vi "TDC_DAQV23_Paralled_muon_temp.vi"(8 "error in (no error)":errorcluster, 9 "stop":bool, 10 "save data":bool=TRUE, 11 "SMA mode":bool) -> (0 "error out 3":errorcluster, 2 "appended path":path=path "D:/tdc/2017/test_20241012_085406.csv", 3 "rate":dbl=30.96114492240285)   [LabVIEW 2017]
uses:
  gloabal.vi
  <vilib>/Utility/file.llb/Write Delimited Spreadsheet (DBL).vi
  <vilib>/Utility/file.llb/Write Delimited Spreadsheet (I64).vi
panel:
  in  "timeout":dbl=120.0 format="%#_13g"
  in  "GPS":bool
  out "name (unnamed)":string
  out "x+y":u64
  out "ip":string[](array[string])
  out "error out 4":errorcluster
  in  "timeout (ms) 2":i32=10000
  in  "address":string[](array[string])=["192.168.10.23", "192.168.10.22"]
  out "substring 4":string
  out "substring 3":string
  out "hex integer string":string="07E8"
  out "Year":string="2024"
  out "substring 2":string
  out "substring":string
  in  "factor":i32=128
  in  "displayCR":bool=TRUE
  in  "Counter Setting":dbl=100000.0 format="%#_13g"
  in  "replace dat":bool
  in  "append csv":bool=TRUE
  out "number":u32=22
  out "element":string
  out "fine":u64=330 format="%x"
  in  "UDP Config":bool=TRUE
  in  "data  path":path=path "D:/tdc/2017"
  out "cal 2":u64[](graph)
  in  "Thresholds (mV)":u16[](array[numeric])=[580, 580, 580, 580, 600, 600, 600, 600, 580, 580, 600, 600, 600, 600, 600, 600, 580, 580, 600, 600, 600, 600, 600, 600, 580, 580, 600, 600, 600, 600, 600, 600]
  out "error out 2":errorcluster
  in  "display":bool=TRUE
  in  "Thresholds":u16=600
  in  "one key for threshold":bool=TRUE
  in  "RST":bool
  in  "通道数量":i32=64
  out "Cal Table":u32[](array[numeric])=[0, 0, 0, 0, 0, 0, 0, 0, 0, 0, 0, 0, 0, 0, 53560, 53560, 0, 0, 0, 0, 0, 0, 0, 0, 0, 0, 0, 0, 0, 0, 0, 0, 0, 0, 0, 0, 0, 0, 0, 0, 0, 0, 0, 0, 0, 0, 0, 0, 0, 0, 0, 0, 0, 0, 0, 0, 0, 0, 0, 0, 0, 0, 0, 0, 0, 0, 0, 0, 0, 0, 0, 0, 0, 0, 0, 0, 0, 0, 0, 0, 0, 0, 0, 0, 0, 0, 0, 0, 0, 0, 0, 0, 0, 0, 0, 0, 0, 0, 0, 0, 0, 0, 0, 0, 0, 0, 0, 0, 0, 0, 0, 0, 0, 0, 0, 0, 0, 0, 53560, 53560, 0, 0, 0, 0, 0, 0, 0, 0]
  in  "channel for cal":i32=61
  out "channel number":u64
  out "Calibration Counter":i32=53569
  out "cal":u32[](graph)
  out "error out":errorcluster
  in  "filename":string="test"
  in  "Events":i32=110000 min=1
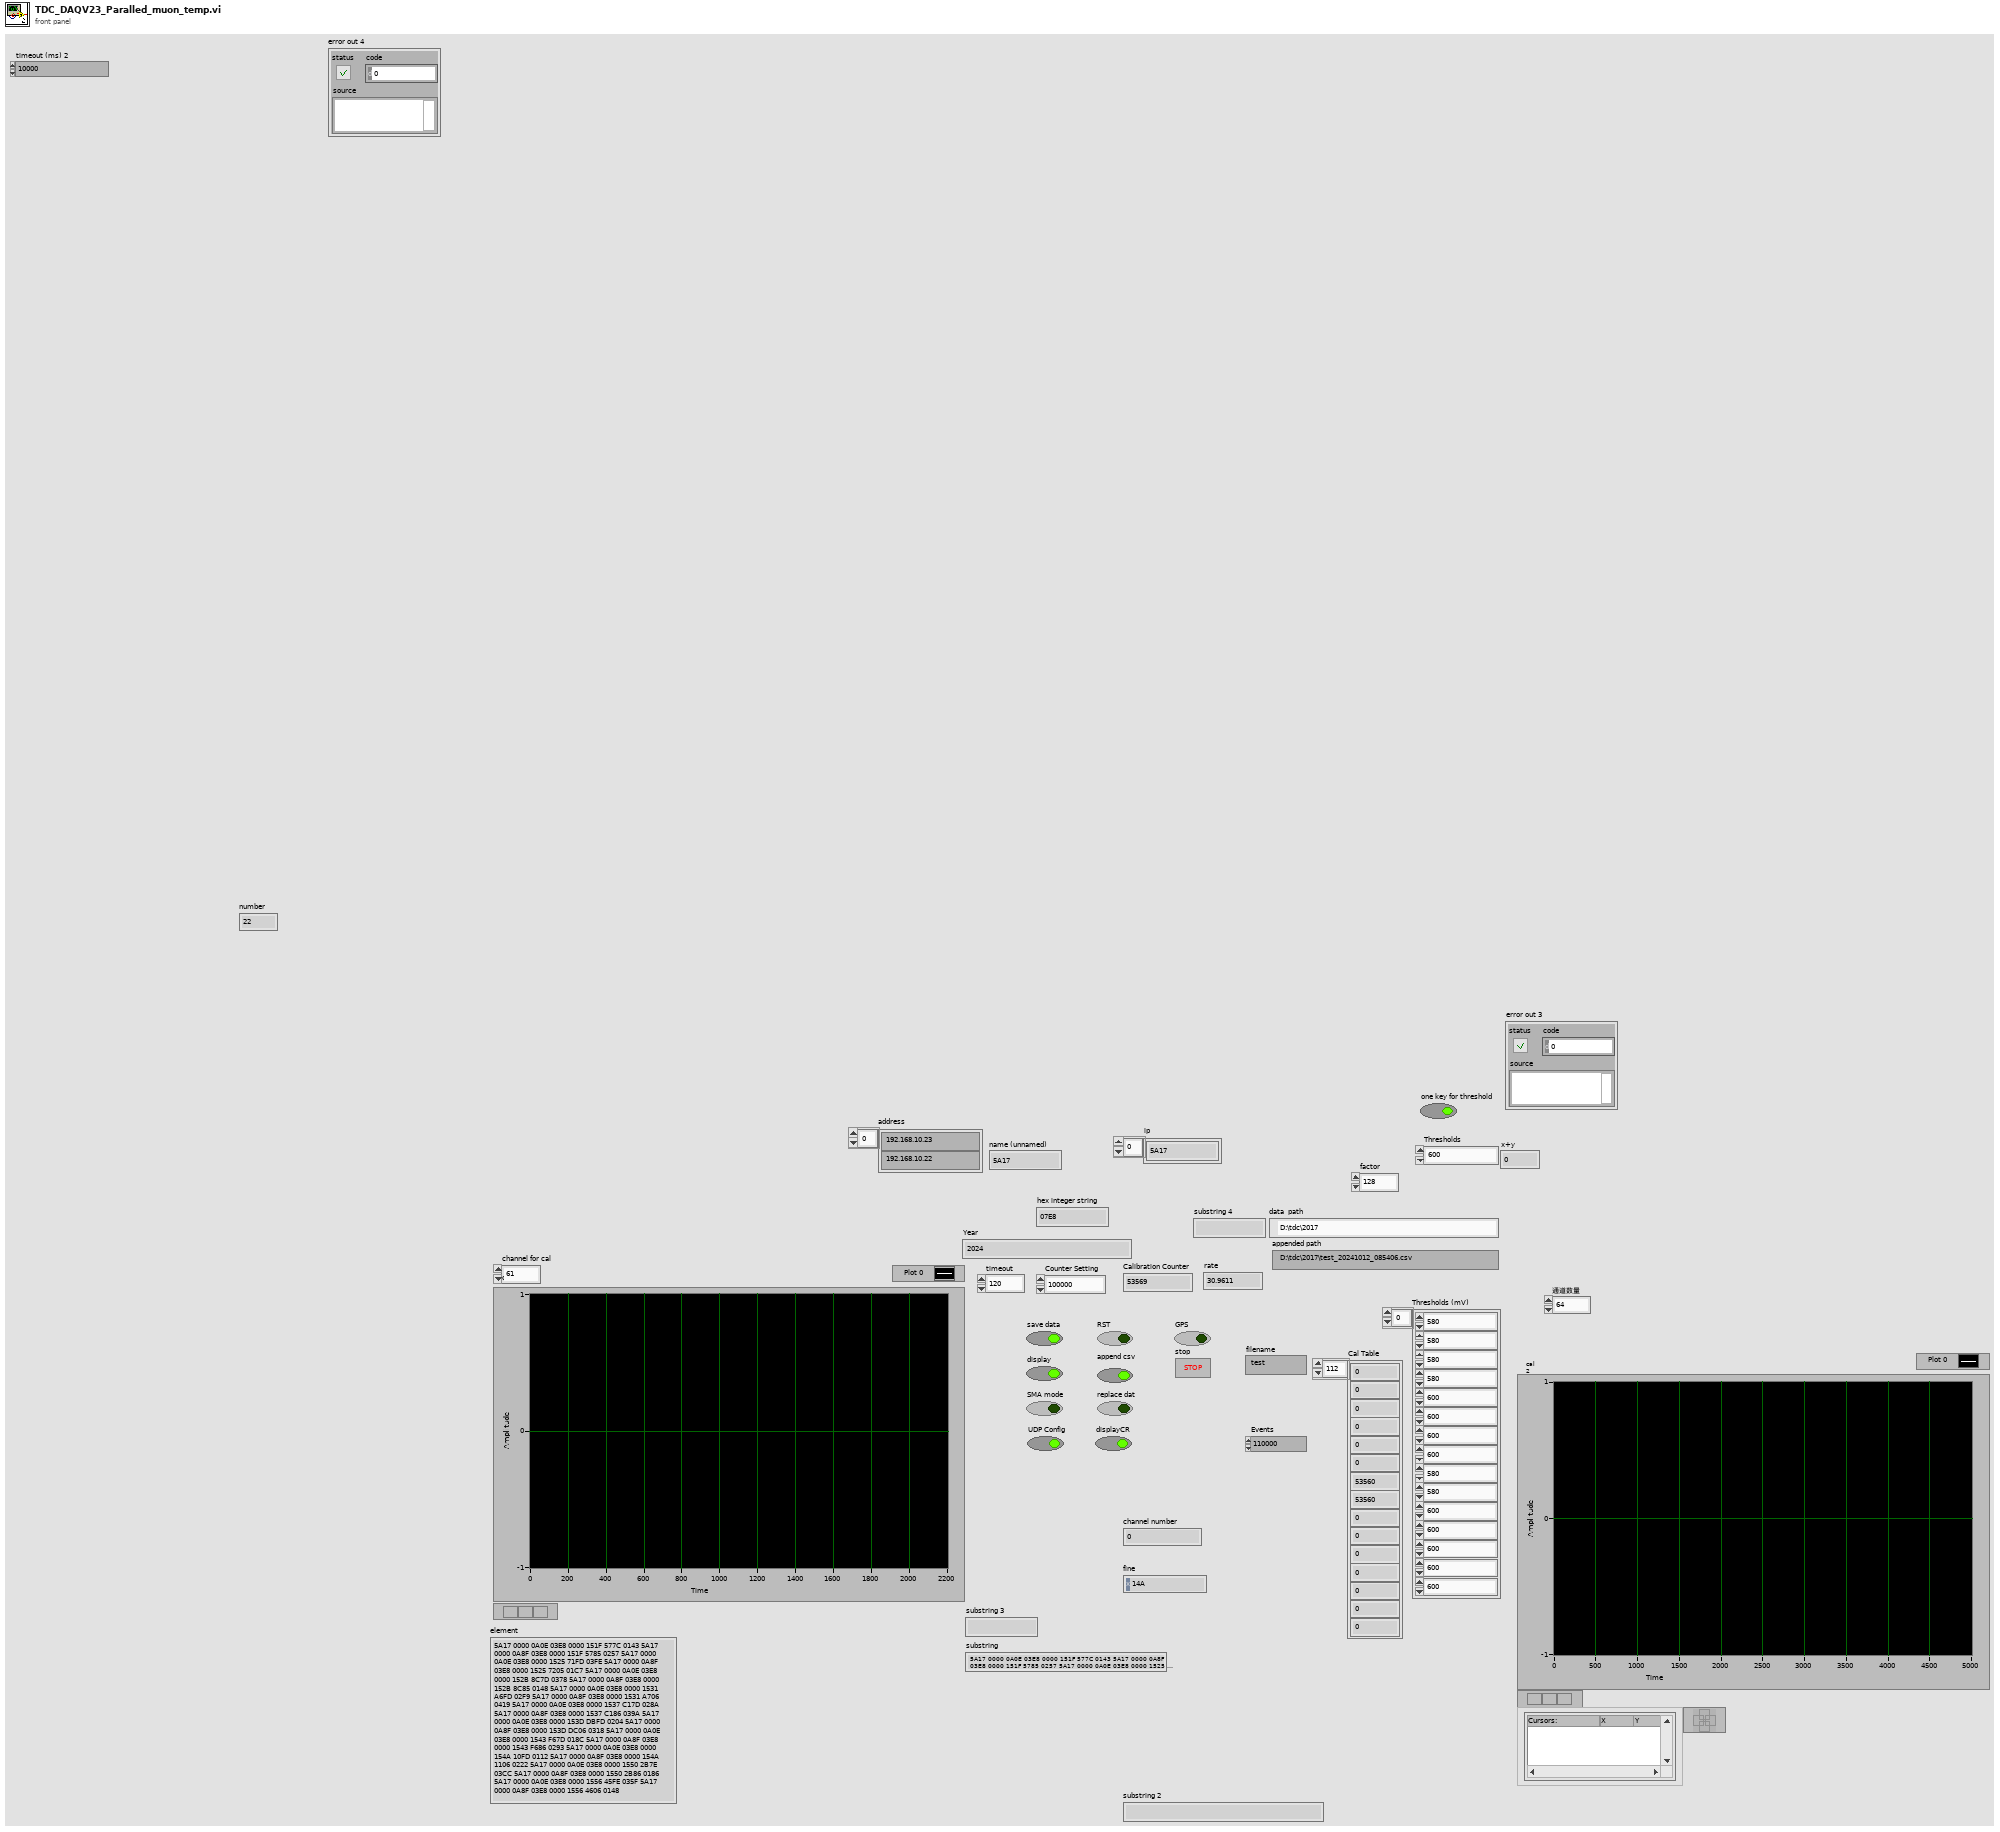
[diagram p1: front panel]
types:
  T1 = enum16{"open", "replace", "create", "open or create", "replace or create", "replace or create with confirmation"}
  T2 = enum16{"big-endian, network order", "native, host order", "little-endian"}
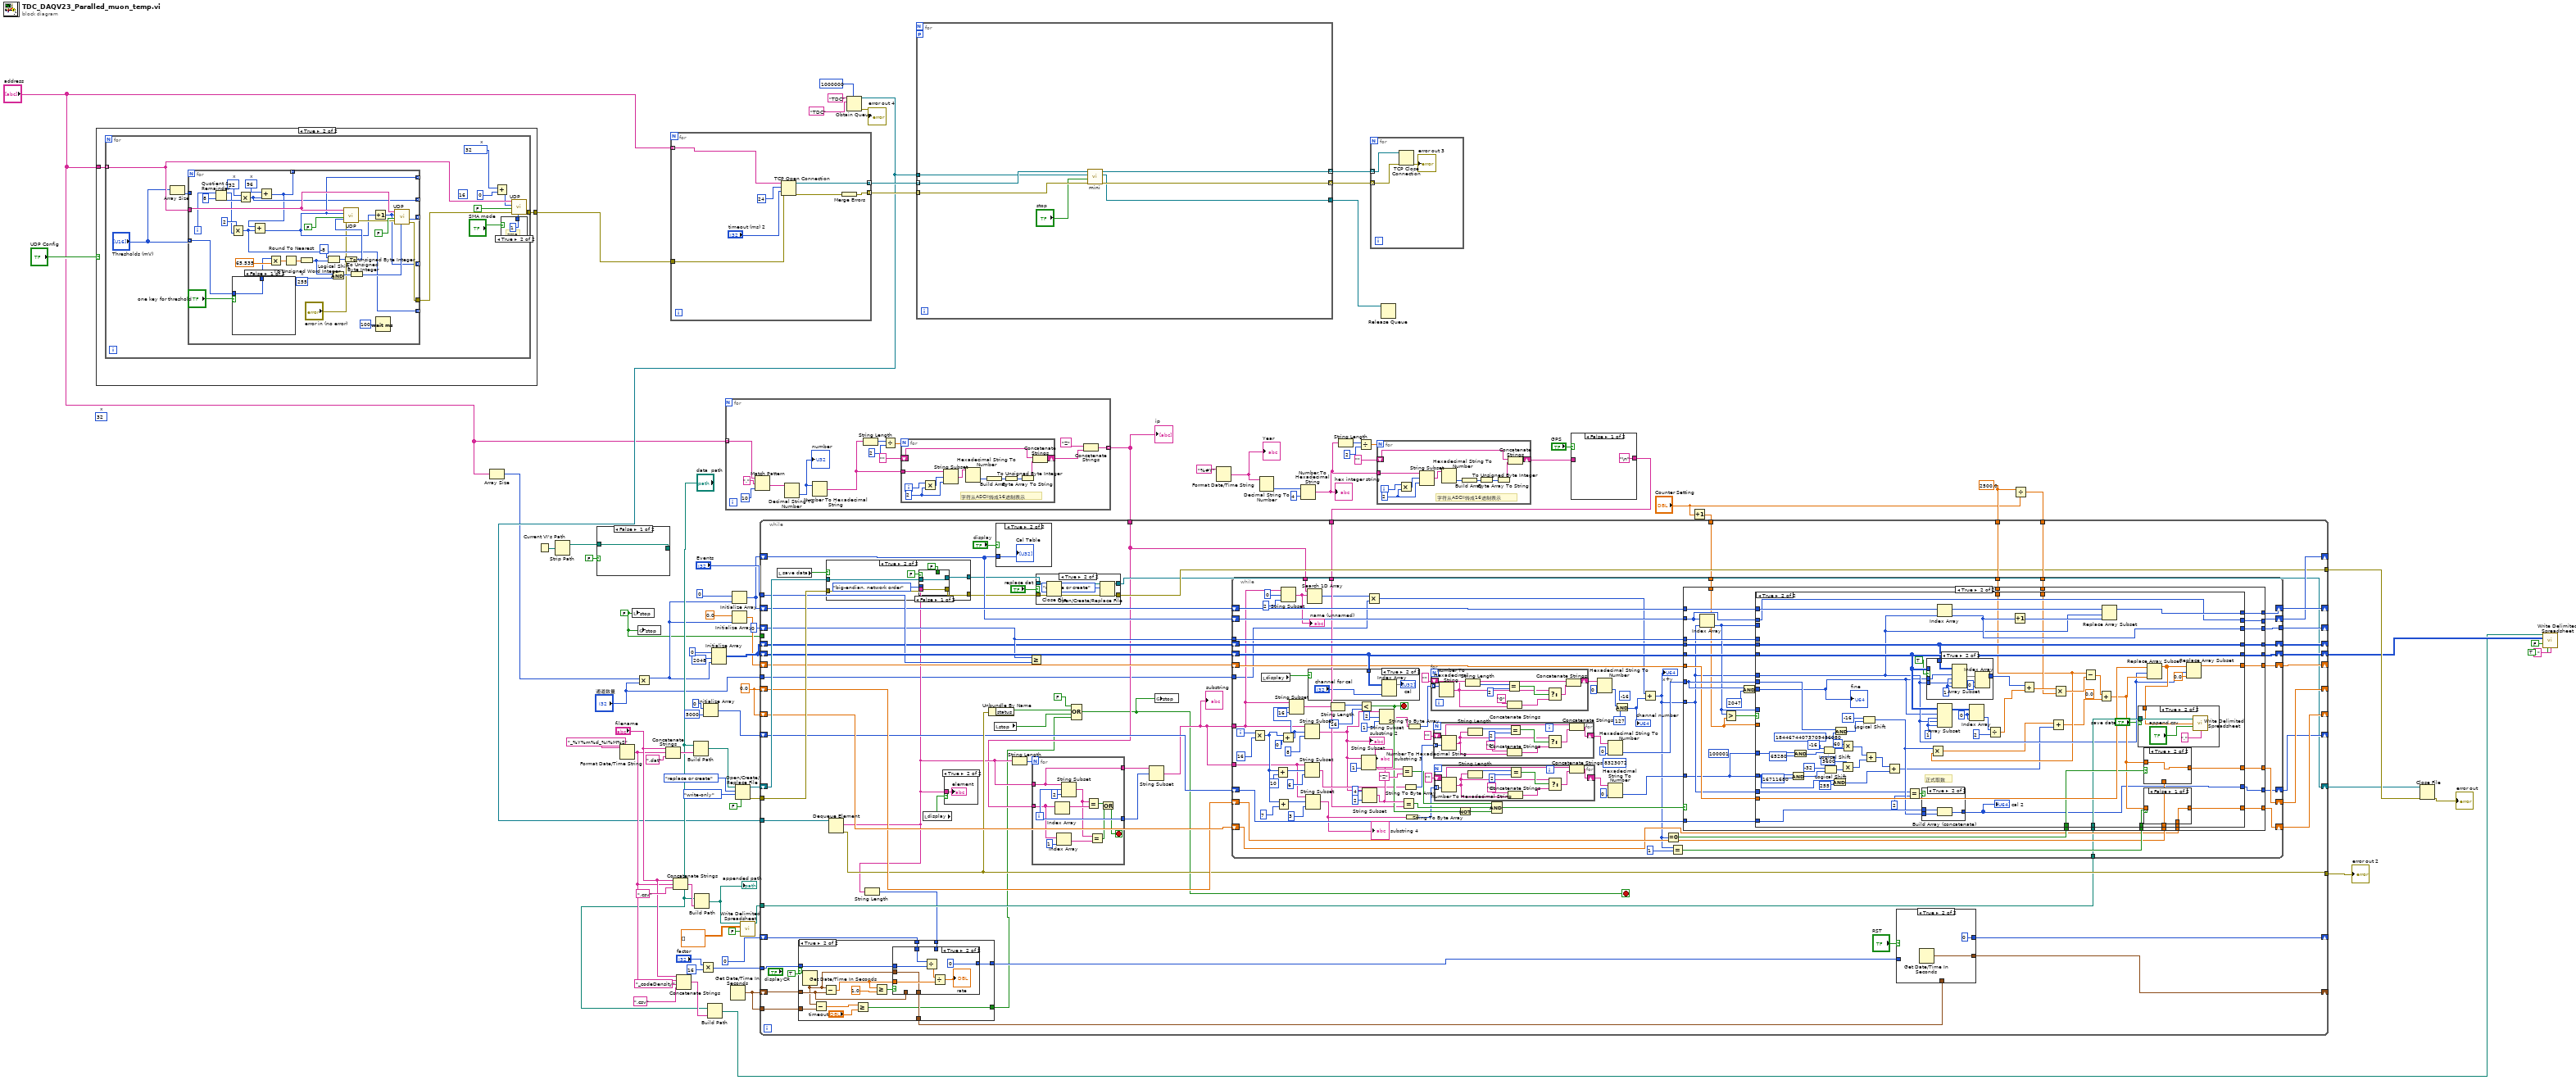
[diagram p0: block diagram]
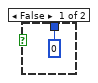
[diagram p4: hidden frame]
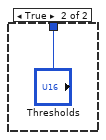
[diagram p5: hidden frame]
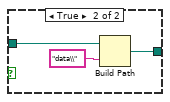
[diagram p6: hidden frame]
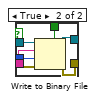
[diagram p9: hidden frame]
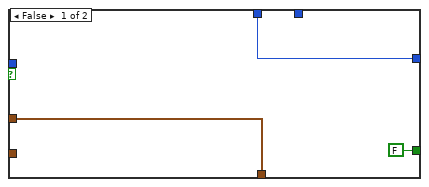
[diagram p11: hidden frame]
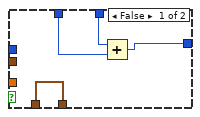
[diagram p12: hidden frame]
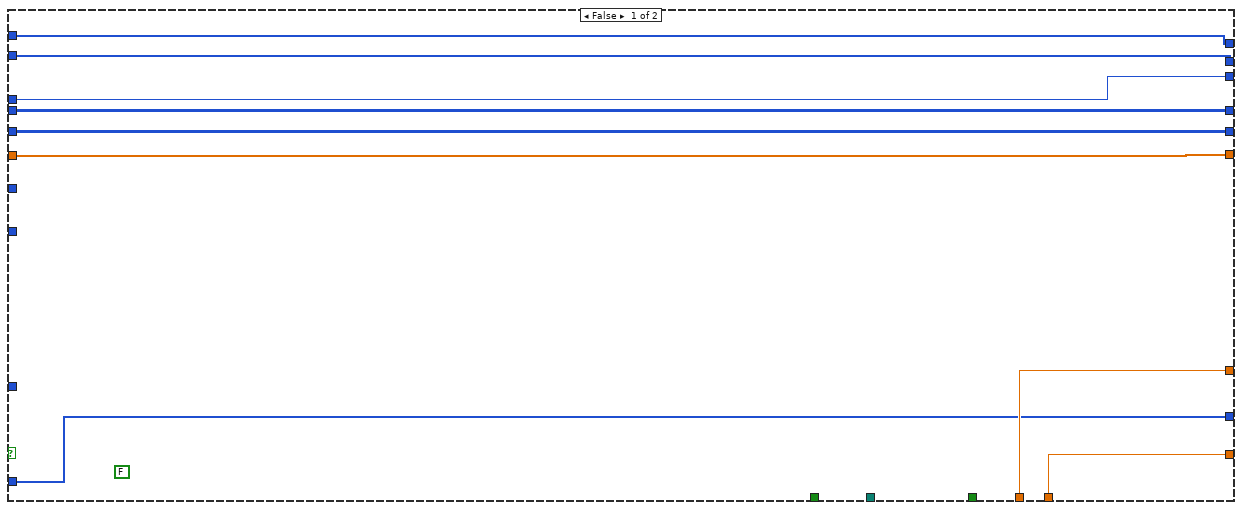
[diagram p16: hidden frame]
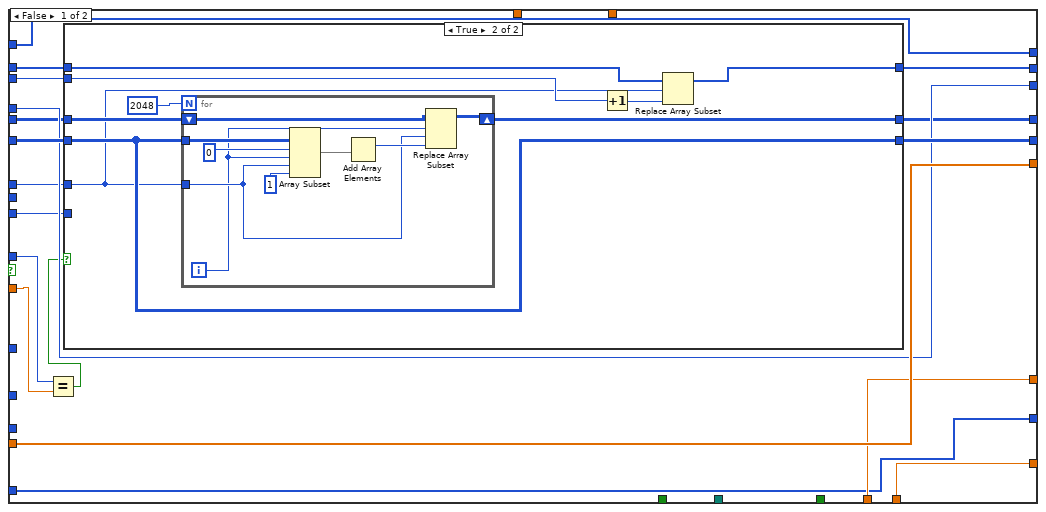
[diagram p17: hidden frame]
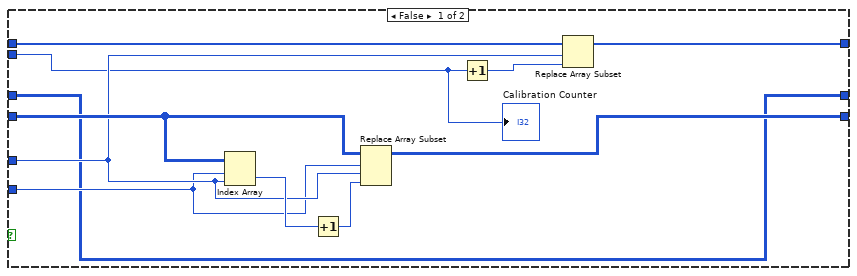
[diagram p18: hidden frame]
diagram:
  w40 = 2500.0 ("x")
  (unwired) u16 32  # x
  w3 = FALSE ("stop")
  w64 = 0.0
  n1 = case shown="True" "UDP Config" {
    tunnel: "address" -> [_ w87]
    tunnel: [_ w86] -> w13
    frame False {
    }
    frame True {
      n2 = for {
        tunnel: w87 -> [w98] mode=indexing
        tunnel: [w95] -> w86
        (unwired) u32 16 ("Address")
        w89 = u16 32  # x
        n3 = Array Size(array="Thresholds (mV)") -> (size(s)=w92:i32)
        n4 = for {
          tunnel: w98 -> [w128]
          tunnel: "Thresholds (mV)" -> [w114] mode=indexing
          tunnel: [w122] -> _ mode=indexing
          tunnel: [w117] -> w96
          tunnel: w92 -> [_]
          tunnel: [w108] -> _ mode=indexing
          tunnel: [w107] -> _ mode=indexing
          tunnel: [w106] -> _ mode=indexing
          tunnel: [w105] -> _ mode=indexing
          tunnel: [w104] -> _ mode=indexing
          i -> [w109]
          w110 = u16 96  # x
          w111 = u16 32  # x
          w124 = u16 255  # x
          n5 = Quotient & Remainder(x=w109, y=8) -> (x-y*floor(x/y)=w103:i32, floor(x/y)=w112:i32)
          n6 = Multiply(x=2, y=w103) -> (x*y=w104:i32)
          n7 = case shown="False" "one key for threshold" {
            tunnel: [w134 "Thresholds"] -> w115
            tunnel: w114 -> [w134 _]
            frame False {
            }
            frame True {
            }
          }
          n8 = Multiply(x=w111, y=w112) -> (x*y=w106:i32)
          n9 = Add(x=w110, y=w106) -> (x+y=w105:i32)
          n10 = Add(x=w105, y=w104) -> (x+y=w108:i32)
          n11 = Multiply(x=w115, y=65.535) -> (x*y=w131:dbl)
          n12 = Round To Nearest(number=w131) -> (nearest integer value=w129:dbl)
          n13 = To Unsigned Word Integer(number=w129) -> (unsigned 16bit integer=w119:u16)
          n14 = Logical Shift(y=i16 -8, x=w119) -> (x << y=w126:u16)
          n15 = And(x=w119, y=w124) -> (x .and. y?=w123:u16)
          n16 = To Unsigned Byte Integer(number=w126) -> (unsigned 8bit integer=w125:u8)
          n17 = call "UDP.vi"("In"=w125, "error in (no error)"="error in (no error)", "Read (TRUE)"=FALSE, "Address"=w108, "IP address"=w128) -> ("error out"=w118:errorcluster)  [unwired: 4 in, 1 out]
          n18 = To Unsigned Byte Integer(number=w123) -> (unsigned 8bit integer=w121:u8)
          n19 = Increment(x=w108) -> (x+1=w107:i32)
          n20 = Wait (ms)(milliseconds to wait=u32 100) -> ()  [unwired: 1 out]
          n21 = call "UDP.vi"("In"=w121, "error in (no error)"=w118, "Read (TRUE)"=FALSE, "Address"=w107, "IP address"=w128) -> ("error out"=w117:errorcluster, "Out"=w122:u8)  [unwired: 4 in]
        }
        n22 = Add(x=w89, y=u32 0 ("Address")) -> (x+y=w88:u32)
        n23 = case shown="True" "SMA mode" {
          tunnel: [u8 0 ("In") u8 1 ("In")] -> w94
          frame False {
          }
          frame True {
            # "sma"
          }
        }
        n24 = call "UDP.vi"("In"=w94, "error in (no error)"=w96, "Read (TRUE)"=FALSE, "Address"=w88, "IP address"=w98) -> ("error out"=w95:errorcluster)  [unwired: 4 in, 1 out]
      }
    }
  }
  n25 = Array Size(array="address") -> (size(s)=w8:i32)
  n26 = Current VI's Path() -> (path=w80:path)
  n27 = Strip Path(path=w80) -> (stripped path=w79:path)  [unwired: 1 out]
  n28 = case shown="False" FALSE {
    tunnel: w79 -> [w136 w138]
    tunnel: [w136 w137] -> _
    frame False {
    }
    frame True {
      n29 = Build Path(base path=w138, name or relative path="data\\") -> (appended path=w137:path)
    }
  }
  n30 = Format Date/Time String(time format string (%c)="_%Y%m%d_%I%M%S") -> (date/time string=w57:string)  [unwired: 2 in]
  n31 = local write "stop"(w3) -> ()
  n32 = Multiply(x=w8, y="通道数量") -> (x*y=w10:i32)
  n33 = global write "gloabal.vi" "stop"(w3) -> ()
  n34 = Concatenate Strings("filename", w57, ".dat") -> (w78:string)
  n35 = for {
    tunnel: "address" -> [w144] mode=indexing
    tunnel: [w143] -> w22 mode=indexing
    tunnel: [w141] -> w21 mode=indexing
    tunnel: w13 -> [w140]
    n36 = TCP Open Connection(address=w144, remote port or service name=u16 24 ("port"), timeout ms (60000)="timeout (ms) 2", error in (no error)=w140) -> (connection ID=w143:refnum<k5>, error out=w142:errorcluster)  [unwired: 1 in]
    n37 = Merge Errors(w142) -> (w141:errorcluster)
  }
  n38 = Concatenate Strings("filename", w57, ".csv") -> (w66:string)
  n39 = Concatenate Strings("filename", w57, "_codeDensity" ("string"), ".csv") -> (w54:string)
  n40 = Build Path(base path="data  path", name or relative path=w78) -> (appended path=w77:path)
  n41 = Build Path(base path="data  path", name or relative path=w66) -> (appended path=w2:path)
  "appended path" <- w2
  n42 = Multiply(x="factor", y=16) -> (x*y=w33:i32)
  n43 = Initialize Array(u32 0 ("element"), 5000 ("dimension size")) -> (w45:u32[])
  n44 = Build Path(base path="data  path", name or relative path=w54) -> (appended path=w51:path)
  n45 = Initialize Array(u32 0 ("element"), 2048 ("dimension size"), w10) -> (w63:u32[][])
  n46 = for {
    tunnel: [w148] -> w9 mode=indexing
    tunnel: "address" -> [w147] mode=indexing
    n47 = Match Pattern(string=w147, regular expression="." ("search string"), offset (0)=10) -> (after substring=w152:string)  [unwired: 3 out]
    n48 = Decimal String To Number(string=w152) -> (number=w151:i32)  [unwired: 2 in, 1 out]
    "number" <- w151
    n49 = Number To Hexadecimal String(2:w151) -> (0:w150:string)  [unwired: 1 in]
    n50 = String Length(string=w150) -> (length=w157:i32)
    n51 = Divide(x=w157, y=2) -> (x/y=w158:dbl)
    n52 = for {
      N: w158 -> [_]
      shift-right: [w170] -> w149
      shift-left: "" ("format string") -> [w169]
      tunnel: w150 -> [w160]
      i -> [w168]
      w162 = 2 ("y")
      # "字符从ASCII转成16进制表示"
      n53 = Multiply(x=w168, y=w162) -> (x*y=w161:i32)
      n54 = String Subset(string=w160, offset (0)=w161, length (rest)=w162) -> (substring=w163:string)
      n55 = Hexadecimal String To Number(string=w163) -> (number=w167:u32)  [unwired: 2 in, 1 out]
      n56 = Build Array(w167) -> (w166:u32[])
      n57 = To Unsigned Byte Integer(number=w166) -> (unsigned 8bit integer=w165:u8[])
      n58 = Byte Array To String(unsigned byte array=w165) -> (string=w164:string)
      n59 = Concatenate Strings(w169, w164) -> (w170:string)
    }
    n60 = Concatenate Strings("Z", w149) -> (w148:string)
  }
  "ip" <- w9
  n61 = Get Date/Time In Seconds() -> (seconds since 1Jan1904=w1:timestamp)
  n62 = Initialize Array(u32 0 ("element"), w10) -> (w65:u32[])
  n63 = Initialize Array(0.0, w10) -> (w47:dbl[])
  n64 = Open/Create/Replace File(file path (use dialog)=w77, operation (0:open)=T1."replace or create", access (0:read/write)=enum16{"read/write", "read-only", "write-only"}."write-only", disable buffering (F)=FALSE) -> (refnum out=w82:refnum<file>, error out=w81:errorcluster)  [unwired: 2 in, 1 out]
  n65 = call-poly <vilib>:"Write Delimited Spreadsheet.vi"("file path (dialog if empty)"=w2, "2D data"=dbl[][] [], "append to file? (new file:F)"=FALSE) -> ("new file path (Not A Path if cancelled)"=w61:path)  [unwired: 11 in, 1 out]
  n66 = Obtain Queue(max queue size (-1, unlimited)=1000000, name (unnamed)="TDC", element data type="TDC" ("name (unnamed)")) -> (queue out=w12:refnum<queue>, error out=→"error out 4":errorcluster)  [unwired: 2 in, 1 out]
  n67 = for {
    tunnel: w22 -> [w177] mode=indexing
    tunnel: w21 -> [w176] mode=indexing
    tunnel: [w175] -> w20 mode=indexing
    tunnel: [w174] -> w19 mode=indexing
    workers-P: _ -> [_]
    tunnel: w12 -> [w173]
    tunnel: [w172] -> w14
    n68 = call "mini.vi"("error in (no error)"=w176, "stop"="stop", "queue out 2"=w173, "connection ID 2"=w177) -> ("error out 3"=w174:errorcluster, "queue out"=w172:refnum<queue>, "connection ID"=w175:refnum<k5>)  [unwired: 5 in]
  }
  n69 = Format Date/Time String(time format string (%c)="%#Y") -> (date/time string=w30:string)  [unwired: 2 in]
  "Year" <- w30
  n70 = Decimal String To Number(string=w30) -> (number=w29:i32)  [unwired: 2 in, 1 out]
  n71 = Number To Hexadecimal String(1:i16 4 ("width (-)"), 2:w29) -> (0:w23:string)
  "hex integer string" <- w23
  n72 = String Length(string=w23) -> (length=w25:i32)
  n73 = Divide(x=w25, y=2) -> (x/y=w26:dbl)
  n74 = for {
    tunnel: w20 -> [w180] mode=indexing
    tunnel: w19 -> [w179] mode=indexing
    n75 = TCP Close Connection(connection ID=w180, error in (no error)=w179) -> (error out=→"error out 3":errorcluster)  [unwired: 1 in, 1 out]
  }
  n76 = for {
    N: w26 -> [_]
    shift-right: [w191] -> w5
    shift-left: "" ("format string") -> [w190]
    tunnel: w23 -> [w181]
    i -> [w189]
    w183 = 2 ("y")
    # "字符从ASCII转成16进制表示"
    n77 = Multiply(x=w189, y=w183) -> (x*y=w182:i32)
    n78 = String Subset(string=w181, offset (0)=w182, length (rest)=w183) -> (substring=w184:string)
    n79 = Hexadecimal String To Number(string=w184) -> (number=w188:u32)  [unwired: 2 in, 1 out]
    n80 = Build Array(w188) -> (w187:u32[])
    n81 = To Unsigned Byte Integer(number=w187) -> (unsigned 8bit integer=w186:u8[])
    n82 = Byte Array To String(unsigned byte array=w186) -> (string=w185:string)
    n83 = Concatenate Strings(w190, w185) -> (w191:string)
  }
  n84 = Release Queue(queue=w14) -> ()  [unwired: 2 in, 3 out]
  n85 = case shown="False" "GPS" {
    tunnel: w5 -> [_ w193]
    tunnel: ["\n" ("format string") w193] -> w4
    frame False {
    }
    frame True {
    }
  }
  n86 = Increment(x="Counter Setting") -> (x+1=w36:dbl)
  n87 = Divide(x=w40, y="Counter Setting") -> (x/y=w39:dbl)
  n88 = while {
    tunnel: w81 -> [w252]
    tunnel: [w227] -> w48
    tunnel: [w212] -> w74
    shift-right: [w249] -> w52
    shift-left: w63 -> [w250]
    shift-right: [w236] -> _
    shift-left: w47 -> [w248]
    tunnel: "Events" -> [w247]
    shift-right: [w246] -> _
    shift-left: w65 -> [w245]
    shift-right: [w244] -> _
    shift-left: u32 0 ("element") -> [w243]
    shift-right: [w242] -> _
    shift-left: w65 -> [w229]
    shift-right: [w241] -> _
    shift-left: w64 -> [w238]
    shift-right: [w240] -> _
    shift-left: w64 -> [w239]
    shift-right: [w231] -> _
    shift-left: w63 -> [w237]
    tunnel: w61 -> [w223]
    shift-right: [w235] -> _
    shift-left: 0 -> [w206]
    shift-right: [w233] -> _
    shift-left: w1 -> [w232]
    tunnel: w3 -> [_]
    tunnel: w12 -> [w228]
    shift-right: [w224] -> _
    shift-left: w45 -> [w225]
    tunnel: w9 -> [w199]
    tunnel: w40 -> [w218]
    tunnel: w39 -> [w217]
    shift-right: [w211] -> w38
    shift-left: w82 -> [w251]
    tunnel: w36 -> [w210]
    tunnel: w33 -> [w203]
    tunnel: w4 -> [w200]
    tunnel: "通道数量" -> [w198]
    tunnel: w1 -> [w194]
    stop <- w196 stop-if-true
    n89 = local read "save data"() -> (w205:bool)
    n90 = Dequeue Element(queue=w228) -> (element=w216:string, error out=w227:errorcluster)  [unwired: 2 in, 2 out]
    n91 = case shown="True" w205 {
      tunnel: w252 -> [w254 w263]
      tunnel: w251 -> [w255 w262]
      tunnel: w216 -> [_ w259]
      tunnel: [w255 w258] -> w215
      tunnel: [w254 w257] -> w213
      frame False {
      }
      frame True {
        n92 = case shown="False" FALSE {
          tunnel: w263 -> [w264 w272]
          tunnel: w262 -> [w265 w271]
          tunnel: T2."big-endian, network order" ("byte order (0:big-endian, network order)") -> [_ w270]
          tunnel: FALSE ("prepend array or string size? (T)") -> [_ w269]
          tunnel: w259 -> [_ w268]
          tunnel: [w265 w267] -> w258
          tunnel: [w264 w266] -> w257
          frame False {
          }
          frame True {
            n93 = Write to Binary File(file (use dialog)=w271, data=w268, error in=w272, 5:w269, 9:w270) -> (refnum out=w267:refnum<file>, error out=w266:errorcluster)  [unwired: 1 in, 1 out]
          }
        }
      }
    }
    n94 = String Length(string=w216) -> (length=w207:i32)
    n95 = case shown="True" TRUE {
      tunnel: w232 -> [w295 w306]
      tunnel: [w295 w307] -> w209
      tunnel: w206 -> [w294 w305]
      tunnel: w207 -> [_ w304]
      tunnel: [w294 w303] -> w208
      tunnel: w203 -> [_ w302]
      tunnel: [FALSE w299] -> w195
      tunnel: w194 -> [_ w298]
      frame False {
      }
      frame True {
        n96 = Get Date/Time In Seconds() -> (seconds since 1Jan1904=w297:timestamp)
        n97 = Subtract(x=w297, y=w298) -> (x-y=w296:dbl)
        n98 = Subtract(x=w297, y=w306) -> (x-y=w301:dbl)
        n99 = Greater Or Equal?(x=w296, y="timeout") -> (x >= y?=w299:bool)
        n100 = Greater Or Equal?(x=w301, y=1.0) -> (x >= y?=w309:bool)
        n101 = case shown="True" w309 {
          tunnel: w301 -> [_ w320]
          tunnel: w297 -> [_ w318]
          tunnel: [w313 w318] -> w307
          tunnel: w306 -> [w313 _]
          tunnel: w305 -> [w312 w315]
          tunnel: w304 -> [w311 _]
          tunnel: [w310 0] -> w303
          tunnel: w302 -> [_ w314]
          frame False {
            n102 = Add(x=w311, y=w312) -> (x+y=w310:i32)
          }
          frame True {
            n103 = Divide(x=w315, y=w314) -> (x/y=w317:dbl)
            n104 = Divide(x=w317, y=w320) -> (x/y=→"rate":dbl)
          }
        }
      }
    }
    n105 = local read "display"() -> (w204:bool)
    n106 = case shown="True" w204 {
      tunnel: w216 -> [_ w253]
      frame False {
      }
      frame True {
        "element" <- w253
      }
    }
    n107 = Unbundle By Name(w227) -> ("status"=w226:bool)
    n108 = local read "stop"() -> (w197:bool)
    n109 = case shown="True" "display" {
      tunnel: w229 -> [_ w321]
      frame False {
      }
      frame True {
        "Cal Table" <- w321
      }
    }
    n110 = String Length(string=w216) -> (length=w222:i32)
    n111 = Greater Or Equal?(x=w243, y=w247) -> ()  [unwired: 1 out]
    n112 = for {
      N: w222 -> [_]
      tunnel: w216 -> [w290]
      tunnel: [w290] -> w221
      tunnel: [w289] -> w220
      tunnel: w199 -> [w287]
      i -> [w289]
      stop <- w283 stop-if-true
      n113 = Index Array(array=w287) -> (element=w288:string)  [unwired: 1 in]
      n114 = Index Array(array=w287, index=1) -> (element=w285:string)
      n115 = String Subset(string=w290, offset (0)=w289, length (rest)=2 ("length (rest)")) -> (substring=w284:string)
      n116 = Equal?(x=w284, y=w288) -> (x = y?=w291:bool)
      n117 = Equal?(x=w284, y=w285) -> (x = y?=w282:bool)
      n118 = Or(x=w291, y=w282) -> (x .or. y?=w283:bool)
    }
    n119 = case shown="True" "replace dat" {
      tunnel: w215 -> [w274 w280]
      tunnel: [w274 w279] -> w211
      tunnel: w213 -> [w273 w276]
      tunnel: [w273 w275] -> w212
      frame False {
      }
      frame True {
        n120 = Close File(refnum=w280, error in=w276) -> (path=w281:path, error out=w277:errorcluster)
        n121 = Open/Create/Replace File(file path (use dialog)=w281, error in=w277, operation (0:open)=T1."replace or create") -> (refnum out=w279:refnum<file>, error out=w275:errorcluster)  [unwired: 3 in, 1 out]
      }
    }
    n122 = Compound Arithmetic op=OR(FALSE ("x"), w226, w197, w195) -> (w196:bool)
    n123 = String Subset(string=w221, offset (0)=w220) -> (substring=w201:string)  [unwired: 1 in]
    "substring" <- w201
    n124 = global write "gloabal.vi" "stop"(w196) -> ()
    n125 = while {
      tunnel: w201 -> [w333]
      shift-right: [w408] -> w249
      shift-left: w250 -> [w406]
      shift-right: [w404] -> w236
      shift-left: w248 -> [w405]
      shift-right: [w401] -> w246
      shift-left: w245 -> [w400]
      tunnel: [w399] -> w244
      tunnel: w243 -> [w398]
      shift-right: [w396] -> w242
      shift-left: w229 -> [w397]
      shift-right: [w392] -> w241
      shift-left: w238 -> [w390]
      shift-right: [w388] -> w240
      shift-left: w239 -> [w389]
      tunnel: w223 -> [w387]
      shift-right: [w386] -> w231
      shift-left: w237 -> [w355]
      shift-right: [w383] -> w224
      shift-left: w225 -> [w384]
      tunnel: w201 -> [w347]
      tunnel: w218 -> [w362]
      tunnel: w217 -> [w361]
      tunnel: w210 -> [w354]
      tunnel: w200 -> [w341]
      tunnel: w199 -> [w332]
      tunnel: w198 -> [w329]
      i -> [w409]
      stop <- w357 stop-if-true
      (unwired) u64 8323072 ("port")
      (unwired) i16 -16 ("y")
      n126 = Multiply(x=w409, y=16 ("length (rest)")) -> (x*y=w348:i32)
      n127 = local read "display"() -> (w385:bool)
      n128 = Add(x=w348, y=10 ("length (rest)")) -> (x+y=w375:i32)
      n129 = Add(x=w348, y=7 ("length (rest)")) -> (x+y=w350:i32)
      n130 = String Subset(string=w333, offset (0)=0, length (rest)=2 ("length (rest)")) -> (substring=w326:string)
      "name (unnamed)" <- w326
      n131 = Add(x=w348, y=0 ("length (rest)")) -> (x+y=w360:i32)
      n132 = String Subset(string=w333, offset (0)=w360, length (rest)=16 ("y")) -> (substring=w358:string)
      n133 = String Subset(string=w333, offset (0)=w360, length (rest)=8 ("length (rest)")) -> (substring=w339:string)
      "substring 2" <- w339
      n134 = String Subset(string=w347, offset (0)=w375, length (rest)=6 ("length (rest)")) -> (substring=w353:string)
      n135 = String Subset(string=w347, offset (0)=w350, length (rest)=3 ("length (rest)")) -> (substring=w336:string)
      "substring 4" <- w336
      n136 = Search 1D Array(1D array=w332, element=w326) -> (index of element=w330:i32)  [unwired: 1 in]
      n137 = case shown="True" w385 {
        tunnel: w406 -> [_ w435]
        frame False {
        }
        frame True {
          n138 = Index Array(array=w435, index (col)="channel for cal") -> (element=→"cal":u32[])  [unwired: 1 in]
        }
      }
      n139 = String Length(string=w358) -> (length=w403:i32)
      n140 = Less?(x=w403, y=16) -> (x < y?=w357:bool)
      n141 = String Subset(string=w339, length (rest)=1 ("length (rest)")) -> (substring=w380:string)  [unwired: 1 in]
      n142 = String Subset(string=w339, offset (0)=4, length (rest)=2 ("length (rest)")) -> (substring=w363:string)
      "substring 3" <- w363
      n143 = Multiply(x=w330, y=w329) -> (x*y=w328:i32)
      n144 = String Subset(string=w339, offset (0)=2, length (rest)=1 ("length (rest)")) -> (substring=w337:string)
      n145 = Equal?(x=w380, y="Z" ("format string")) -> (x = y?=w365:bool)
      n146 = Equal?(x=w363, y=w341) -> (x = y?=w364:bool)
      n147 = String To Byte Array(string=w353) -> (unsigned byte array=w372:u8[])
      n148 = String To Byte Array(string=w336) -> (unsigned byte array=w343:u8[])
      n149 = String To Byte Array(string=w337) -> (unsigned byte array=w411:u8[])
      n150 = for {
        shift-right: [w623] -> w369
        shift-left: "" ("format string") -> [w620]
        tunnel: w411 -> [w624] mode=indexing
        n151 = Number To Hexadecimal String(2:w624) -> (0:w616:string)  [unwired: 1 in]
        n152 = String Length(string=w616) -> (length=w622:i32)
        n153 = Equal?(x=w622, y=2) -> (x = y?=w619:bool)
        n154 = Concatenate Strings("0" ("format string"), w616) -> (w618:string)
        n155 = Select(t=w616, s=w619, f=w618) -> (s? t:f=w615:string)
        n156 = Concatenate Strings(w620, w615) -> (w623:string)
      }
      n157 = for {
        shift-right: [w431] -> w370
        shift-left: "" ("format string") -> [w423]
        tunnel: w372 -> [w432] mode=indexing
        n158 = Number To Hexadecimal String(2:w432) -> (0:w425:string)  [unwired: 1 in]
        n159 = String Length(string=w425) -> (length=w430:i32)
        n160 = Concatenate Strings("0" ("format string"), w425) -> (w427:string)
        n161 = Equal?(x=w430, y=2) -> (x = y?=w428:bool)
        n162 = Select(t=w425, s=w428, f=w427) -> (s? t:f=w424:string)
        n163 = Concatenate Strings(w423, w424) -> (w431:string)
      }
      n164 = for {
        shift-right: [w421] -> w346
        shift-left: "" ("format string") -> [w413]
        tunnel: w343 -> [w422] mode=indexing
        n165 = Number To Hexadecimal String(2:w422) -> (0:w415:string)  [unwired: 1 in]
        n166 = String Length(string=w415) -> (length=w420:i32)
        n167 = Concatenate Strings("0" ("format string"), w415) -> (w417:string)
        n168 = Equal?(x=w420, y=2) -> (x = y?=w418:bool)
        n169 = Select(t=w415, s=w418, f=w417) -> (s? t:f=w414:string)
        n170 = Concatenate Strings(w413, w414) -> (w421:string)
      }
      n171 = Not(x=w357) -> (.not. x?=w356:bool)
      n172 = Compound Arithmetic op=AND(w365, w364, w356) -> (w378:bool)
      n173 = Hexadecimal String To Number(string=w369, default (0uL)=u64 0 ("default (0 U32)")) -> (number=w407:u64)  [unwired: 1 in, 1 out]
      n174 = Hexadecimal String To Number(string=w370, default (0uL)=u64 0 ("default (0 U32)")) -> (number=w368:u64)  [unwired: 1 in, 1 out]
      n175 = Hexadecimal String To Number(string=w346, default (0uL)=u64 0 ("default (0 U32)")) -> (number=w342:u64)  [unwired: 1 in, 1 out]
      n176 = And(x=w407, y=u64 127 ("port")) -> (x .and. y?=w331:u64)
      "channel number" <- w331
      n177 = Add(x=w328, y=w331) -> (x+y=w327:u64)
      "x+y" <- w327
      n178 = Equal To 0?(x=w327) -> (x = 0?=w393:bool)
      n179 = Equal?(x=w327, y=u64 1) -> (x = y?=w391:bool)
      n180 = case shown="True" w378 {
        tunnel: w368 -> [_ w475]
        tunnel: w398 -> [w441 w465]
        tunnel: w406 -> [w444 w474]
        tunnel: [w444 w473] -> w408
        tunnel: [w443 w470] -> w404
        tunnel: w405 -> [w443 w469]
        tunnel: w327 -> [_ w449]
        tunnel: w400 -> [w442 w468]
        tunnel: [w442 w467] -> w401
        tunnel: [w441 w466] -> w399
        tunnel: w397 -> [w440 w464]
        tunnel: [w440 w463] -> w396
        tunnel: w393 -> [_ w462]
        tunnel: w390 -> [w439 w461]
        tunnel: [w439 w460] -> w392
        tunnel: w391 -> [_ w459]
        tunnel: w389 -> [w438 w458]
        tunnel: [w438 w457] -> w388
        tunnel: w355 -> [w437 w455]
        tunnel: [w437 w454] -> w386
        tunnel: w387 -> [_ w453]
        tunnel: w384 -> [w436 w451]
        tunnel: [w436 w450] -> w383
        tunnel: w362 -> [_ w448]
        tunnel: w361 -> [_ w447]
        tunnel: w354 -> [_ w446]
        tunnel: w342 -> [_ w445]
        frame False {
          (unwired) FALSE
        }
        frame True {
          (unwired) 100001 ("y")
          n181 = Index Array(array=w464, index=w449) -> (element=w456:u32)
          n182 = Greater?(x=w456, y=w446) -> (0:w452:bool)
          n183 = And(x=w475, y=u64 2047 ("port")) -> (x .and. y?=w471:u64)
          n184 = case shown="True" w452 {
            tunnel: w475 -> [_ w587]
            tunnel: w474 -> [w493 w573]
            tunnel: [w492 w573] -> w473
            tunnel: w471 -> [w484 w546]
            tunnel: [w491 w557] -> w470
            tunnel: w469 -> [w491 w580]
            tunnel: w465 -> [w489 _]
            tunnel: w449 -> [w487 w555]
            tunnel: w468 -> [w490 w579]
            tunnel: [w490 w578] -> w467
            tunnel: [w489 w576] -> w466
            tunnel: w456 -> [w485 _]
            tunnel: w464 -> [w488 w575]
            tunnel: [w486 w575] -> w463
            tunnel: w462 -> [_ w568]
            tunnel: w461 -> [w483 w567]
            tunnel: [w483 w566] -> w460
            tunnel: w459 -> [_ w565]
            tunnel: w458 -> [w482 w564]
            tunnel: [w482 w563] -> w457
            tunnel: w456 -> [w480 _]
            tunnel: w446 -> [w477 _]
            tunnel: w455 -> [w479 w559]
            tunnel: [w478 w559] -> w454
            tunnel: w453 -> [_ w558]
            tunnel: w451 -> [w476 w552]
            tunnel: [w476 w550] -> w450
            tunnel: w449 -> [_ w547]
            tunnel: w448 -> [_ w544]
            tunnel: w447 -> [_ w545]
            tunnel: w445 -> [_ w539]
            tunnel: w445 -> [_ w527]
            frame False {
              n185 = Equal?(x=w480, y=w477) -> (x = y?=w481:bool)
              n186 = case shown="True" w481 {
                tunnel: w493 -> [w504 w510]
                tunnel: [w502 w510] -> w492
                tunnel: w488 -> [w500 w508]
                tunnel: w487 -> [w499 w505]
                tunnel: [w497 w507] -> w486
                tunnel: w485 -> [w496 w506]
                tunnel: w484 -> [w495 _]
                tunnel: w479 -> [w494 w512]
                tunnel: [w494 w511] -> w478
                frame False {
                  n187 = Index Array(array=w504, index (row)=w495, index (col)=w499) -> (element=w503:u32)
                  n188 = Increment(x=w503) -> (x+1=w501:u32)
                  n189 = Replace Array Subset(array=w504, new element=w501, index (row)=w495, index (col)=w499) -> (w502:u32[][])
                  n190 = Increment(x=w496) -> (x+1=w498:u32)
                  n191 = Replace Array Subset(array=w500, new element=w498, index=w499) -> (w497:u32[])
                  "Calibration Counter" <- w496
                }
                frame True {
                  n192 = for {
                    N: 2048 -> [_]
                    tunnel: w510 -> [w522]
                    tunnel: w505 -> [w515]
                    shift-right: [w517] -> w511
                    shift-left: w512 -> [w518]
                    i -> [w514]
                    n193 = Array Subset(array=w522, index (row)=0 ("索引"), length (row)=w514, index (col)=w515, length (col)=1 ("长度")) -> (w519:u32[][])
                    n194 = Add Array Elements(numeric array=w519) -> (sum=w516:u32)
                    n195 = Replace Array Subset(array=w518, new element=w516, index (row)=w514, index (col)=w515) -> (w517:u32[][])
                  }
                  n196 = Increment(x=w506) -> (x+1=w509:u32)
                  n197 = Replace Array Subset(array=w508, new element=w509, index=w505) -> (w507:u32[])
                }
              }
            }
            frame True {
              (unwired) 0.0 ("x")
              w570 = 0 ("索引 (行)")
              w572 = 1 ("长度")
              # "正式取数"
              n198 = And(x=w527, y=u64 16711680 ("port")) -> (x .and. y?=w536:u64)
              n199 = And(x=w539, y=u64 65280 ("port")) -> (x .and. y?=w542:u64)
              n200 = Logical Shift(y=i16 -16, x=w542) -> (x << y=w533:u64)
              n201 = Logical Shift(y=i16 -32, x=w536) -> (x << y=w535:u64)
              n202 = And(x=w527, y=u64 255 ("port")) -> (x .and. y?=w526:u64)
              n203 = And(x=w587, y=u64 18446744073709486080 ("port")) -> (x .and. y?=w584:u64)
              n204 = Multiply(x=u64 3600, y=w535) -> (x*y=w530:u64)
              n205 = Multiply(x=u64 60, y=w533) -> (x*y=w531:u64)
              n206 = Logical Shift(y=i16 -16, x=w584) -> (x << y=w551:u64)
              n207 = Add(x=w531, y=w530) -> (x+y=w529:u64)
              n208 = Add(x=w529, y=w526) -> (x+y=w523:u64)
              n209 = Equal?(x=w547, y=u32 2) -> (x = y?=w549:bool)
              n210 = case shown="True" w549 {
                tunnel: w552 -> [w588 w591]
                tunnel: w551 -> [_ w590]
                tunnel: [w588 w589] -> w550
                frame False {
                }
                frame True {
                  n211 = Build Array (concatenate)(w591, w590) -> (w589:u64[])
                }
              }
              "cal 2" <- w550
              n212 = case shown="True" TRUE {
                tunnel: [w598 w606] -> w582
                tunnel: w573 -> [_ _]
                tunnel: w555 -> [w603 w604]
                tunnel: w546 -> [w601 w609]
                tunnel: w559 -> [w602 w610]
                frame False {
                  w597 = 0 ("index (row)")
                  w600 = 1 ("长度")
                  n213 = Decrement(x=w603) -> (x-1=w596:u64)
                  n214 = Array Subset(array=w602, index (row)=w601, length (row)=w600, index (col)=w596, length (col)=w600) -> (w599:u32[][])
                  n215 = Index Array(array=w599, index (row)=w597, index (col)=w597) -> (element=w598:u32)
                }
                frame True {
                  w605 = 0 ("index (row)")
                  w608 = 1 ("长度")
                  n216 = Array Subset(array=w610, index (row)=w609, length (row)=w608, index (col)=w604, length (col)=w608) -> (w607:u32[][])
                  n217 = Index Array(array=w607, index (row)=w605, index (col)=w605) -> (element=w606:u32)
                }
              }
              n218 = Multiply(x=w551, y=w544) -> (x*y=w525:dbl)
              n219 = Index Array(array=w579, index=w555) -> (element=w576:u32)
              n220 = Array Subset(array=w573, index (row)=w546, length (row)=w572, index (col)=w555, length (col)=w572) -> (w571:u32[][])
              n221 = Index Array(array=w571, index (row)=w570, index (col)=w570) -> (element=w569:u32)
              n222 = Divide(x=w569, y=u32 2) -> (x/y=w574:dbl)
              n223 = Increment(x=w576) -> (x+1=w577:u32)
              n224 = Add(x=w582, y=w574) -> (x+y=w581:dbl)
              n225 = Add(x=w525, y=w523) -> (x+y=w524:dbl)
              n226 = Multiply(x=w581, y=w545) -> (x*y=w561:dbl)
              n227 = Subtract(x=w544, y=w561) -> (x-y=w543:dbl)
              n228 = Add(x=w543, y=w524) -> (x+y=w562:dbl)
              n229 = Replace Array Subset(array=w579, new element=w577, index=w555) -> (w578:u32[])
              n230 = case shown="True" w568 {
                tunnel: w562 -> [_ w614]
                tunnel: [w613 w614] -> w566
                tunnel: w567 -> [w613 _]
                frame False {
                }
                frame True {
                }
              }
              n231 = case shown="False" w565 {
                tunnel: [w611 w612] -> w563
                tunnel: w564 -> [w611 _]
                tunnel: w562 -> [_ w612]
                frame False {
                }
                frame True {
                }
              }
              n232 = Replace Array Subset(array=w580, new element=w562, index=w555) -> (w556:dbl[])
              n233 = case shown="True" "save data" {
                tunnel: w558 -> [_ w595]
                tunnel: w556 -> [_ w593]
                frame False {
                }
                frame True {
                  n234 = call-poly <vilib>:"Write Delimited Spreadsheet.vi"("file path (dialog if empty)"=w595, "1D data"=w593, "append to file? (new file:F)"="append csv", "delimiter (\\t)"="," ("delimiter (\\t)")) -> ()  [unwired: 10 in, 2 out]
                }
              }
              n235 = Replace Array Subset(array=w556, new element=0.0 ("new element/subarray"), index=w555) -> (w557:dbl[])
              "fine" <- w546
            }
          }
        }
      }
    }
    n236 = case shown="True" "RST" {
      tunnel: w208 -> [w323 _]
      tunnel: [w323 0] -> w235
      tunnel: [w322 w324] -> w233
      tunnel: w209 -> [w322 _]
      frame False {
      }
      frame True {
        n237 = Get Date/Time In Seconds() -> (seconds since 1Jan1904=w324:timestamp)
      }
    }
  }
  "error out 2" <- w48
  n238 = Close File(refnum=w38, error in=w74) -> (error out=→"error out":errorcluster)  [unwired: 1 out]
  n239 = call-poly <vilib>:"Write Delimited Spreadsheet.vi"("file path (dialog if empty)"=w51, "2D data"=w52, "append to file? (new file:F)"=FALSE, "transpose? (no:F)"=TRUE, "delimiter (\\t)"="," ("delimiter (\\t)")) -> ()  [unwired: 9 in, 2 out]
